vi "SDSU_dacs-volts.vi"(0 "dac":i32, 5 "Table In":string[][](table), 7 "action":enum16{"DAC2VOLT", "VOLT2DAC"}(ring), 9 "input value":dbl format="%.3f") -> (8 "string value":string, 10 "output value":dbl format="%.3f")   [LabVIEW 2016]
panel:
  out "output 1":dbl format="%.6f"
  out "output variable":dbl format="%.2f"
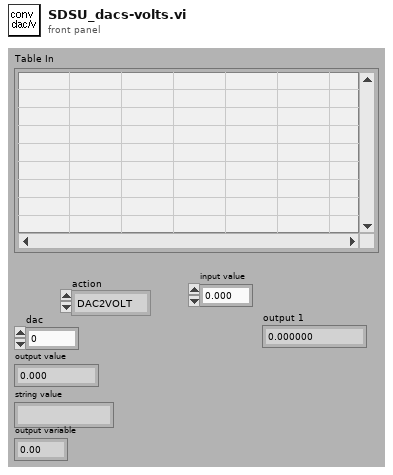
[diagram p1: front panel]
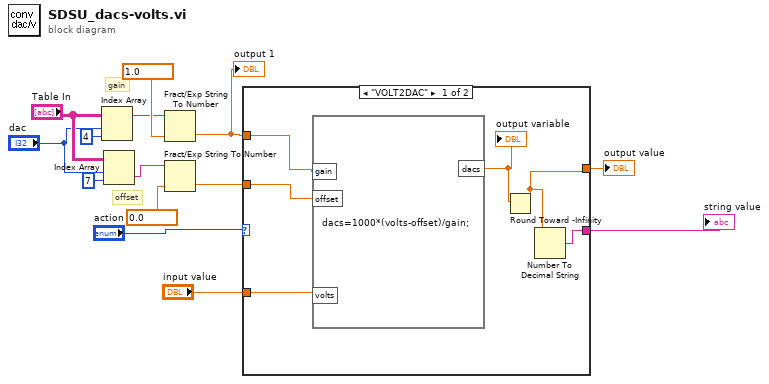
[diagram p0: block diagram]
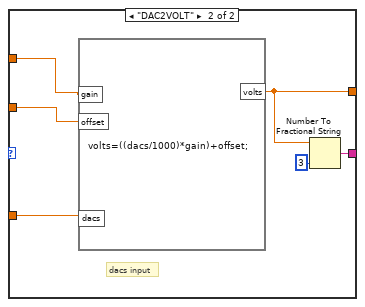
[diagram p2: hidden frame]
diagram:
  # "offset"
  # "gain"
  n1 = Index Array(array="Table In", index (row)="dac", index (col)=4 ("disabled index (col)")) -> (element=w2:string)
  n2 = Index Array(array="Table In", index (row)="dac", index (col)=7 ("disabled index (col)")) -> (element=w8:string)
  n3 = Fract/Exp String To Number(string=w2, default (0 dbl)=1.0) -> (number=w1:dbl)  [unwired: 3 out]
  "output 1" <- w1
  n4 = Fract/Exp String To Number(string=w8, default (0 dbl)=0.0) -> (number=w6:dbl)  [unwired: 3 out]
  n5 = case shown="\"VOLT2DAC\"" "action" {
    tunnel: w1 -> [w20 w26]
    tunnel: w6 -> [w19 w25]
    tunnel: "input value" -> [w18 w24]
    tunnel: [w15 w22] -> w4
    tunnel: [w16 w21] -> w3
    frame "VOLT2DAC" {
      n6 = formula code="dacs=1000*(volts-offset)/gain;"("gain"=w20, "offset"=w19, "volts"=w18) -> ("dacs"=w17:dbl)
      "output variable" <- w17
      n7 = Round Toward -Infinity(1:w17) -> (0:w15:dbl)
      n8 = Number To Decimal String(number=w15) -> (decimal integer string=w16:string)  [unwired: 1 out]
    }
    frame "DAC2VOLT" {
      # "dacs input"
      n9 = formula code="volts=((dacs/1000)*gain)+offset;"("gain"=w26, "offset"=w25, "dacs"=w24) -> ("volts"=w22:dbl)
      n10 = Number To Fractional String(number=w22, precision (6)=i16 3) -> (F-format string=w21:string)  [unwired: 2 out]
    }
  }
  "output value" <- w4
  "string value" <- w3
